vi "HeadingGoodnessAtHeading.vi"(11 "Heading":i32) -> (3 "Heading goodness\nat this heading":sgl)   [LabVIEW 2011]
panel:
  out "Angle in radians":sgl
  out "cos(x)":sgl
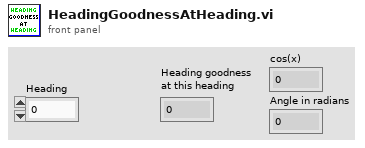
[diagram p1: front panel]
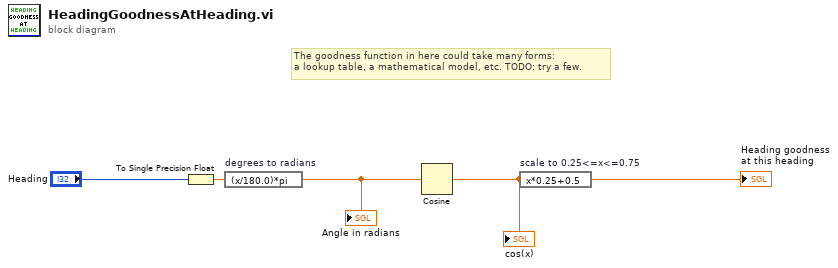
[diagram p0: block diagram]
diagram:
  # "The goodness function in here could take many forms:\na lookup table, a mathematical model, etc. TODO: try a few."
  n1 = To Single Precision Float(number="Heading") -> (single precision float=w5:sgl)
  n2 = expression code="(x/180.0)*pi" "degrees to radians"(w5) -> (w4:sgl)
  "Angle in radians" <- w4
  n3 = Cosine(x=w4) -> (cos(x)=w3:sgl)
  "cos(x)" <- w3
  n4 = expression code="x*0.25+0.5" "scale to 0.25<=x<=0.75"(w3) -> (→"Heading goodness\nat this heading":sgl)
